vi "micro1 pvgen500_P.vi"(0 "FluxStrIn":string, 1 "Numin":i32, 5 "errin":errorcluster, 6 "Data label":string, 8 "tab ref":string[][](array[string]), 10 "ligne à traiter":string[](array[string])) -> (14 "result string":string, 15 "Numout":i32, 19 "errout":errorcluster)   [LabVIEW 2020]
uses:
  VG/VG_DeltaTcell_P.vi
  ZEN8 Semi Auto EMC/OP700/VG/VG_TCellmax.vi
  ZEN8 Semi Auto EMC/OP700/VG/VG_TCellmin.vi
  VG/IS30%_P.vi
  VG/VG_VCellMin70_P.vi
  VG/VG_VCellMax70_P.vi
  VG/VG_VCellMin30_P.vi
  VG/VG_VCellMax30_P.vi
  VG/VG_DeltaVcell_P.vi
  <vilib>/regexp/Match Regular Expression.xnode
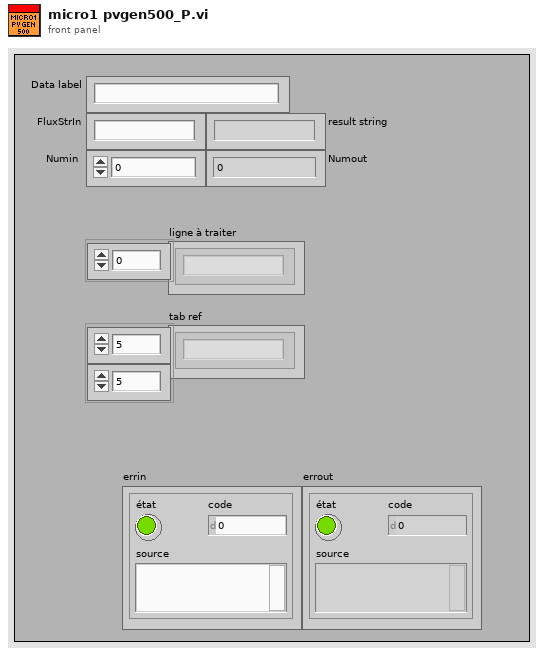
[diagram p1: front panel]
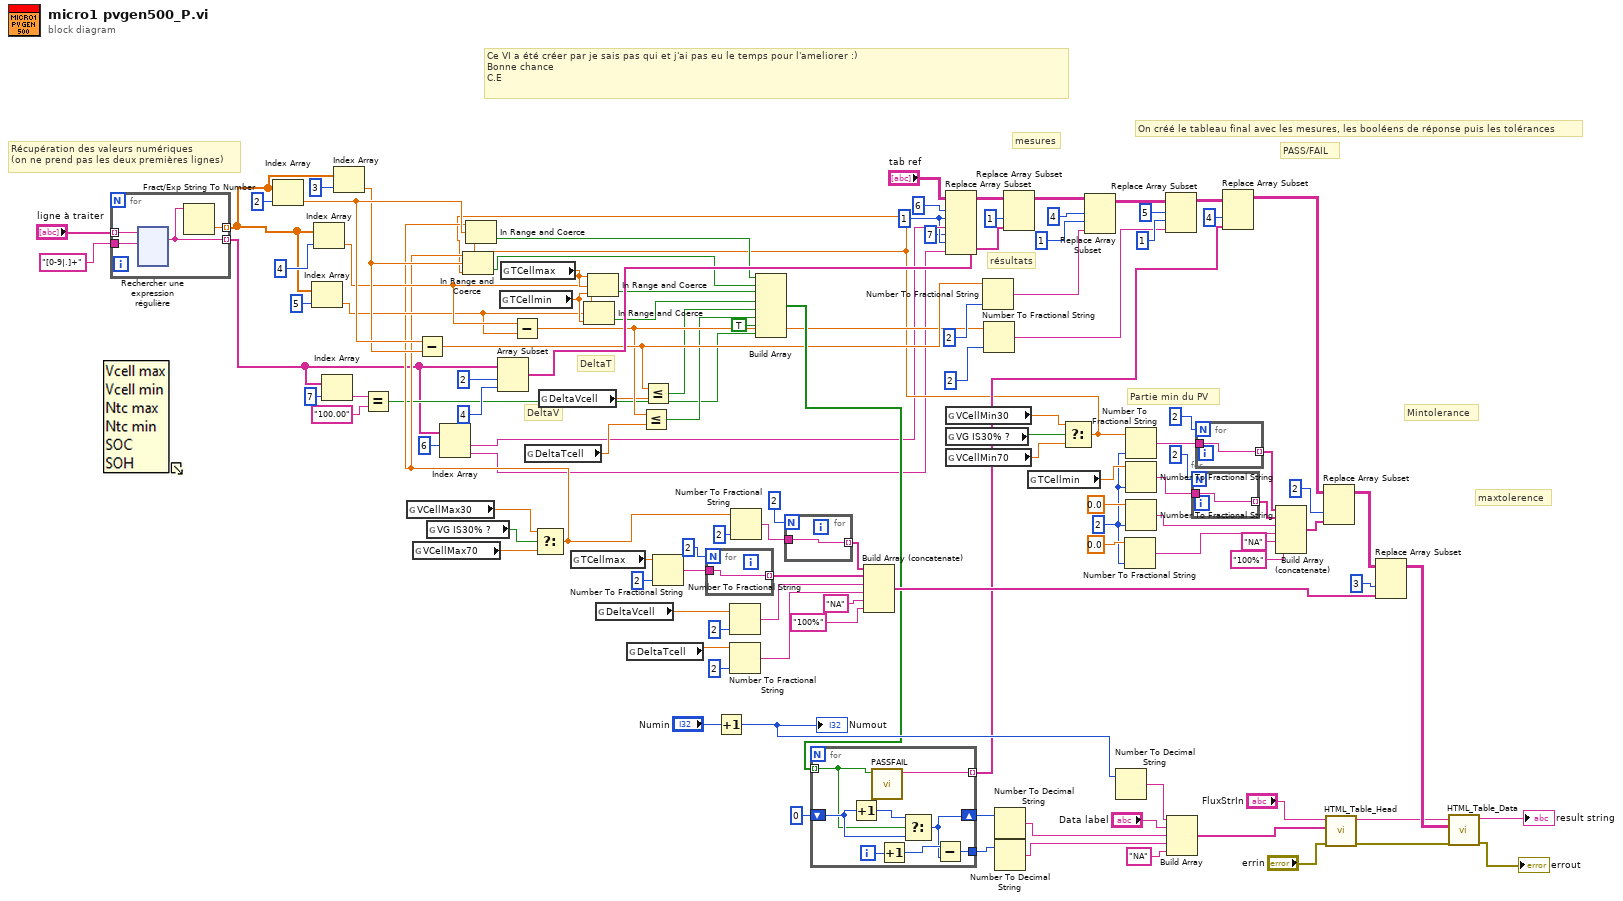
[diagram p0: block diagram]
diagram:
  w3 = 1 ("disabled index (col)")
  w49 = 2
  # "Ce VI a été créer par je sais pas qui et j'ai pas eu le temps pour l'ameliorer :)\nBonne chance\nC.E"
  # "DeltaV"
  # "DeltaT"
  # "Partie min du PV"
  # "Récupération des valeurs numériques\n(on ne prend pas les deux premières lignes)"
  # "On créé le tableau final avec les mesures, les booléens de réponse puis les tolérances"
  # "maxtolerence"
  # "Mintolerance"
  # "mesures"
  # "PASS/FAIL"
  # "résultats"
  n1 = for {
    tunnel: "ligne à traiter" -> [w122] mode=indexing
    tunnel: "[0-9|.]+" ("expression régulière") -> [w121]
    tunnel: [w120] -> w15 mode=indexing
    tunnel: [w119] -> w6 mode=indexing
    n2 = xnode "Rechercher une expression régulière"("input string"=w122, "regular expression"=w121) -> ("whole match"=w119:string)  [unwired: 4 in, 4 out]
    n3 = Fract/Exp String To Number(string=w119) -> (number=w120:dbl)  [unwired: 3 in, 1 out]
  }
  n4 = Index Array(array=w15, index=2 ("indice")) -> (element=w34:dbl)
  n5 = Index Array(array=w15, index=5 ("indice")) -> (element=w31:dbl)
  n6 = Index Array(array=w15, index=4 ("longueur")) -> (element=w32:dbl)
  n7 = Index Array(array=w6, index=7) -> (element=w13:string)
  n8 = Index Array(array=w15, index=3 ("indice")) -> (element=w33:dbl)
  n9 = Equal?(x=w13, y="100.00") -> (x = y?=w12:bool)
  n10 = global read "VG_VCellMax30_P.vi" "VCellMax30"() -> (w29:dbl)
  n11 = global read "VG_VCellMax70_P.vi" "VCellMax70"() -> (w28:dbl)
  n12 = Subtract(x=w34, y=w33) -> (x-y=w47:dbl)
  n13 = global read "IS30%_P.vi" "VG IS30% ?"() -> (w30:bool)
  n14 = Index Array(array=w6, index #1=6 ("index")) -> (element #1=w4:string, element #2=w1:string)  [unwired: 1 in]
  n15 = Array Subset(array=w6, index=2 ("indice"), length=4 ("longueur")) -> (w91:string[])
  n16 = global read "VG_TCellmin.vi" "TCellmin"() -> (w36:dbl)
  n17 = global read "VG_TCellmax.vi" "TCellmax"() -> (w37:dbl)
  n18 = Subtract(x=w32, y=w31) -> (x-y=w45:dbl)
  n19 = global read "VG_DeltaTcell_P.vi" "DeltaTcell"() -> (w46:dbl)
  n20 = Select(t=w29, s=w30, f=w28) -> (s? t:f=w24:dbl)
  n21 = global read "VG_DeltaVcell_P.vi" "DeltaVcell"() -> (w22:dbl)
  n22 = global read "VG_TCellmax.vi" "TCellmax"() -> (w66:dbl)
  n23 = In Range and Coerce(upper limit=w37, x=w31, lower limit=w36) -> (In Range?=w35:bool)  [unwired: 1 out]
  n24 = In Range and Coerce(upper limit=w37, x=w32, lower limit=w36) -> (In Range?=w54:bool)  [unwired: 1 out]
  n25 = global read "VG_DeltaVcell_P.vi" "DeltaVcell"() -> (w21:dbl)
  n26 = global read "VG_DeltaTcell_P.vi" "DeltaTcell"() -> (w65:dbl)
  n27 = Less Or Equal?(x=w45, y=w46) -> (x <= y?=w44:bool)
  n28 = Less Or Equal?(x=w47, y=w22) -> (x <= y?=w42:bool)
  n29 = Number To Fractional String(number=w66, precision (6)=i16 2 ("précision (6)")) -> (F-format string=w62:string)  [unwired: 2 in]
  n30 = for {
    N: 2 -> [_]
    tunnel: w62 -> [w237]
    tunnel: [w237] -> w61 mode=indexing
  }
  n31 = Increment(x="Numin") -> (x+1=w104:i32)
  "Numout" <- w104
  n32 = Number To Fractional String(number=w21, precision (6)=i16 2 ("précision (6)")) -> (F-format string=w64:string)  [unwired: 2 in]
  n33 = Number To Fractional String(number=w65, precision (6)=i16 2 ("précision (6)")) -> (F-format string=w63:string)  [unwired: 2 in]
  n34 = Number To Fractional String(number=w24, precision (6)=i16 2 ("précision (6)")) -> (F-format string=w67:string)  [unwired: 2 in]
  n35 = for {
    N: 2 -> [_]
    tunnel: w67 -> [w238]
    tunnel: [w238] -> w76 mode=indexing
  }
  n36 = Build Array (concatenate)(w76, w61, w64, w63, "NA" ("element"), "100%" ("element")) -> (w118:string[])
  n37 = Replace Array Subset(array="tab ref", new element #1=w4, index (row) #1=6 ("disabled index (row)"), index (col) #1=w3, new element #2=w1, index (row) #2=7 ("disabled index (row)"), index (col) #2=w3) -> (w8:string[][])
  n38 = global read "VG_VCellMin30_P.vi" "VCellMin30"() -> (w25:dbl)
  n39 = global read "IS30%_P.vi" "VG IS30% ?"() -> (w27:bool)
  n40 = global read "VG_VCellMin70_P.vi" "VCellMin70"() -> (w26:dbl)
  n41 = Number To Fractional String(number=w47, precision (6)=i16 2) -> (F-format string=w81:string)  [unwired: 2 in]
  n42 = Number To Fractional String(number=w45, precision (6)=i16 2) -> (F-format string=w78:string)  [unwired: 2 in]
  n43 = Replace Array Subset(array=w8, new element=w91, index (col)=1 ("indice désactivé (col)")) -> (w85:string[][])  [unwired: 1 in]
  n44 = global read "VG_TCellmin.vi" "TCellmin"() -> (w59:dbl)
  n45 = Select(t=w25, s=w27, f=w26) -> (s? t:f=w23:dbl)
  n46 = In Range and Coerce(upper limit=w24, x=w33, lower limit=w23) -> (In Range?=w39:bool)  [unwired: 1 out]
  n47 = In Range and Coerce(upper limit=w24, x=w34, lower limit=w23) -> (In Range?=w41:bool)  [unwired: 1 out]
  n48 = Build Array(w41, w39, w54, w35, w42, w44, TRUE ("element"), w12) -> (w53:bool[])
  n49 = for {
    tunnel: w53 -> [w239] mode=indexing
    tunnel: [w240] -> w89 mode=indexing
    shift-right: [w242] -> w106
    shift-left: 0 -> [w245]
    tunnel: [w241] -> w107
    i -> [w244]
    n50 = Increment(x=w245) -> (x+1=w246:i32)
    n51 = call <userlib>:"PASSFAIL.vi"("E"=w239) -> ("S"=w240:string)  [unwired: 10 in]
    n52 = Increment(x=w244) -> (x+1=w243:i32)
    n53 = Select(t=w246, s=w239, f=w245) -> (s? t:f=w242:i32)
    n54 = Subtract(x=w243, y=w242) -> (x-y=w241:i32)
  }
  n55 = Number To Decimal String(number=w106) -> (decimal integer string=w108:string)  [unwired: 1 in]
  n56 = Number To Decimal String(number=w107) -> (decimal integer string=w109:string)  [unwired: 1 in]
  n57 = Replace Array Subset(array=w85, new element=w81, index (row)=4 ("disabled index (row)"), index (col)=1 ("disabled index (col)")) -> (w83:string[][])
  n58 = Number To Decimal String(number=w104) -> (decimal integer string=w93:string)  [unwired: 1 in]
  n59 = Number To Fractional String(number=0.0 ("nombre"), precision (6)=w49) -> (F-format string=w55:string)  [unwired: 2 in]
  n60 = Number To Fractional String(number=w23, precision (6)=w49) -> (F-format string=w60:string)  [unwired: 2 in]
  n61 = Number To Fractional String(number=w59, precision (6)=w49) -> (F-format string=w52:string)  [unwired: 2 in]
  n62 = Number To Fractional String(number=0.0 ("nombre"), precision (6)=w49) -> (F-format string=w57:string)  [unwired: 2 in]
  n63 = Replace Array Subset(array=w83, new element=w78, index (row)=5 ("disabled index (row)"), index (col)=1 ("disabled index (col)")) -> (w82:string[][])
  n64 = Build Array(w93, "Data label", w108, w109, "NA" ("élément")) -> (w96:string[])
  n65 = for {
    N: 2 -> [_]
    tunnel: w52 -> [w247]
    tunnel: [w247] -> w51 mode=indexing
  }
  n66 = for {
    N: 2 -> [_]
    tunnel: w60 -> [w248]
    tunnel: [w248] -> w73 mode=indexing
  }
  n67 = Replace Array Subset(array=w82, new element=w89, index (col)=4 ("indice désactivé (col)")) -> (w112:string[][])  [unwired: 1 in]
  n68 = Build Array (concatenate)(w73, w51, w57, w55, "NA" ("element"), "100%" ("element")) -> (w117:string[])
  n69 = Replace Array Subset(array=w112, new element=w117, index (col)=2 ("indice désactivé (col)")) -> (w114:string[][])  [unwired: 1 in]
  n70 = call "HTML_Table_Head.vi"("entrée d'erreur (pas d'erreur)"="errin", "Tableau"=w96, "chaîne en entrée"="FluxStrIn") -> ("sortie d'erreur"=w95:errorcluster, "result string"=w94:string)  [unwired: 7 in]
  n71 = Replace Array Subset(array=w114, new element=w118, index (col)=3 ("indice désactivé (col)")) -> (w113:string[][])  [unwired: 1 in]
  n72 = call "HTML_Table_Data.vi"("entrée d'erreur (pas d'erreur)"=w95, "Tableau"=w113, "chaîne en entrée"=w94) -> ("sortie d'erreur"=→"errout":errorcluster, "result string"=→"result string":string)  [unwired: 7 in]
